vi "Write Minimum Pane Size.vi"(5 "Minimum Pane Size":T1, 9 "Pane in":refnum<class "Pane.lvclass">) -> (3 "Pane out":refnum<class "Pane.lvclass">)   [LabVIEW 2014, in "Pane.lvclass"]
uses:
  Pane.lvclass
  <vilib>/Utility/miscctls.llb/LVPointTypeDef.ctl
  Pane.lvclass/Pane.ctl
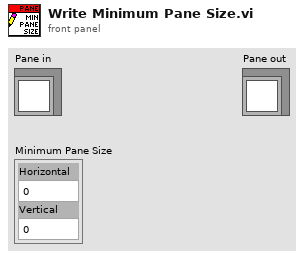
[diagram p1: front panel]
types:
  T1 = typedef "LVPointTypeDef.ctl" = cluster{"Horizontal":i16, "Vertical":i16}
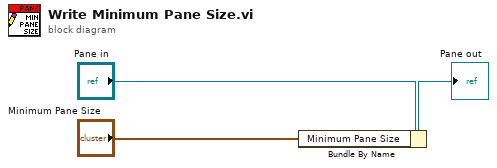
[diagram p0: block diagram]
diagram:
  n1 = Bundle By Name(cluster="Pane in", "Minimum Pane Size"="Minimum Pane Size") -> (→"Pane out":refnum<class "Pane.lvclass">)
